vi "Filepaths global.vi"() -> ()   [LabVIEW 2010]
panel:
  in  "Sim images":path
  in  "Project dir":path
  in  ".ini path":path
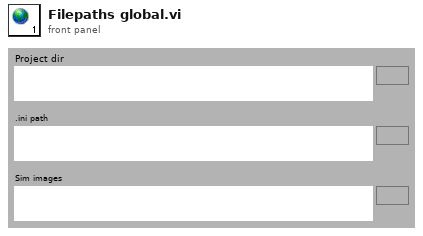
[diagram p1: front panel]
diagram:
